vi "Execute.vi"(8 "error in":errorcluster, 11 "Denuder STEP":refnum<class "Denuder STEP.lvclass">) -> (0 "error out":errorcluster, 1 "Next Step?":bool, 2 "MSG":string, 3 "Denuder STEP out":refnum<class "Denuder STEP.lvclass">)   [LabVIEW 2014, in "Denuder STEP.lvclass"]
uses:
  Denuder STEP.lvclass
  <vilib>/ActorFramework/Message Enqueuer/Message Enqueuer.lvclass
  Controller/Messages/Change Denuder State/Change Denuder State MSG.lvclass
  reusable/Sequence/STEPS/STEP.lvclass/STEP.ctl
  Controller/Messages/Change Denuder State/Change Denuder State MSG.lvclass/Change Denuder State MSG.ctl
  <vilib>/ActorFramework/Message Enqueuer/Message Enqueuer.lvclass/Message Enqueuer.ctl
  reusable/Sequence/STEPS/Read Obj.vi
  Controller/Messages/Change Denuder State/Write denude_.vi
  <vilib>/ActorFramework/Message Priority Queue/Priority Enqueue.vi
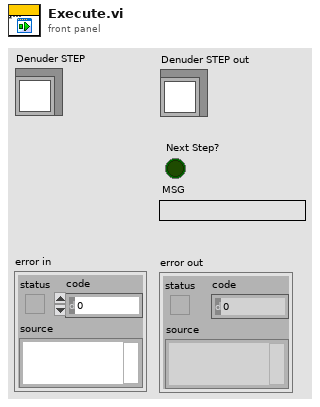
[diagram p1: front panel]
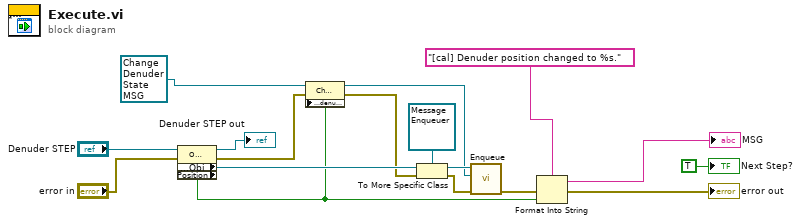
[diagram p0: block diagram]
diagram:
  n1 = property class="O2 Valve"(reference="Denuder STEP", error in="error in") -> (reference out=→"Denuder STEP out":refnum<class "Denuder STEP.lvclass">, error out=w3:errorcluster, "Accessors:Obj"=w17:refnum<class>, "Position"=w6:bool)
  n2 = property class="Change Denuder State MSG"(reference=refnum<class "Change Denuder State MSG.lvclass"> refnum ("Controller:Change Denuder State MSG"), error in=w3, "Accessors:denude_"=w6) -> (reference out=w5:refnum<class "Change Denuder State MSG.lvclass">, error out=w2:errorcluster)
  n3 = To More Specific Class(target class=refnum<class "Message Enqueuer.lvclass"> refnum ("Message Enqueuer in"), reference=w17, error in=w2) -> (specific class reference=w14:refnum<class "Message Enqueuer.lvclass">, error out=w15:errorcluster)
  n4 = call <vilib>:"Enqueue.vi"("error in (no error)"=w15, "Message"=w5, "Message Enqueuer in"=w14) -> ("error out"=w12:errorcluster)  [unwired: 7 in, 1 out]
  n5 = Format Into String(format string="[cal] Denuder position changed to %s.", error in=w12, w6) -> (resulting string=→"MSG":string, error out=→"error out":errorcluster)  [unwired: 1 in]
  "Next Step?" <- TRUE ("Next Step?")
